vi "String to numeric.vi"(5 "Array":string[](array[string])) -> (2 "Array 2":dbl[](array[numeric]))   [LabVIEW 2017]
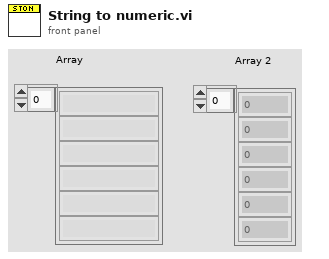
[diagram p1: front panel]
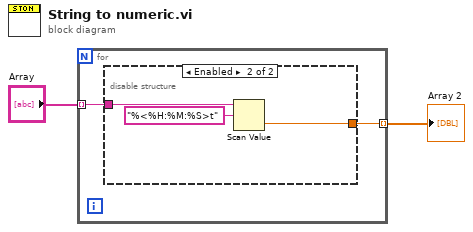
[diagram p0: block diagram]
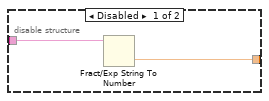
[diagram p2: hidden frame]
diagram:
  n1 = for {
    tunnel: "Array" -> [w4] mode=indexing
    tunnel: [w3] -> w1 mode=indexing
    n2 = disable-structure shown="Enabled" {
      disable-tunnel: w4 -> [w6 w9]
      disable-tunnel: [w5 w7] -> w3
      frame Disabled {
        n3 = Fract/Exp String To Number(string=w6) -> (number=w5:dbl)  [unwired: 3 in, 1 out]
      }
      frame Enabled {
        n4 = Scan Value(string=w9, format string="%<%H:%M:%S>t") -> (value=w7:dbl)  [unwired: 1 in, 1 out]
      }
    }
  }
  "Array 2" <- w1
